vi "Read_DSS_Monitors.vi"(8 "error in (no error)":errorcluster) -> (0 "error out":errorcluster, 2 "Monitor 2":string[][](array[string]), 3 "monitor 1":string[][](array[string]))   [LabVIEW 2010]
doc: "This VI implements the routine for reading the Monitors placed at the OpenDSS simulation. the monitors data is droped on .csv files in the system's temporary folder. this routine looks for those files and delivers a matrix (String) for each monitor.\n\nCreted by Davis montenegro\n06-29-2017"
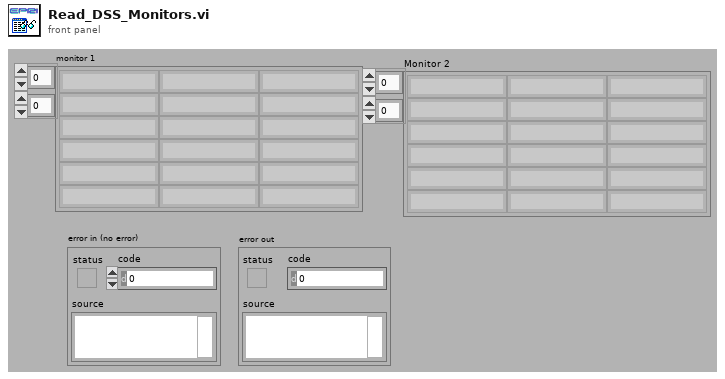
[diagram p1: front panel]
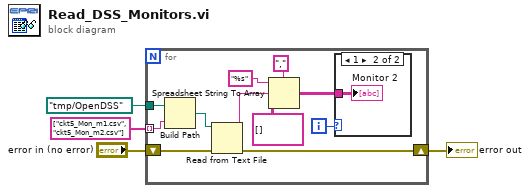
[diagram p0: block diagram]
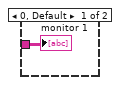
[diagram p2: hidden frame]
diagram:
  n1 = for {
    tunnel: path "/tmp/OpenDSS" ("file (use dialog)") -> [w13]
    shift-right: [w15] -> w4
    shift-left: "error in (no error)" -> [w12]
    tunnel: string[] ["ckt5_Mon_m1.csv", "ckt5_Mon_m2.csv"] -> [w11] mode=indexing
    i -> [w6]
    n2 = Build Path(base path=w13, name or relative path=w11) -> (appended path=w14:path)
    n3 = Read from Text File(file (use dialog)=w14, error in=w12) -> (text=w7:string, error out=w15:errorcluster)  [unwired: 2 in, 2 out]
    n4 = Spreadsheet String To Array(delimiter (Tab)=",", format string="%s", spreadsheet string=w7, array type (2D Dbl)=string[][] []) -> (array=w5:string[][])
    n5 = case shown="1" w6 {
      tunnel: w5 -> [w16 w17]
      frame 0, Default {
        "monitor 1" <- w16
      }
      frame 1 {
        "Monitor 2" <- w17
      }
    }
  }
  "error out" <- w4
